vi "NI 5772 (AC) - TIS Mode Enabled (FPGA)Original.vi"() -> ()   [LabVIEW 2020]
doc: "Example Description:\nThis example demonstrates how to enable Time Interleaved Sampling with the NI 5772 adapter module to achieve a sampling rate of 1.6GS/s. This example continuously acquires records of analog input data from the NI 5772 adapter module. It allows you to select an AI channel, trigger type, and record size. This VI must be compiled before it is run. \n\nRunning the VI:\nThis VI must be run from the NI 5772 - Getting Started (Host).vi. Refer to the host VI documentation for steps regarding running and configuring the FPGA VI. \n\nExecution Steps:\nRefer to the Block Diagram of this VI for execution comments."
uses:
  D:/Program_Files/Labview2018/LabVIEW 2020/examples/FlexRIO/IO Modules/NI 5772/NI 5772 (AC) - TIS Mode Enabled/Controls/AI Trigger Type.ctl
  D:/Program_Files/Labview2018/LabVIEW 2020/examples/FlexRIO/IO Modules/NI 5772/NI 5772 (AC) - TIS Mode Enabled/Controls/Aquire State.ctl
  <vilib>/Platform/TimedLoop/XDataNode/timing_clust.ctl
  <vilib>/Platform/TimedLoop/XDataNode/nitl_modes.ctl
  <vilib>/Platform/TimedLoop/XDataNode/wakeup.ctl
  <vilib>/rvi/Emulation/niFpgaGetClockAttributes.vi
  <vilib>/rvi/Emulation/niFpgaSctlEmulationGetInTimedLoop.vi
  <vilib>/rvi/Emulation/niFpgaEmulationReportErrorSimple.vi
  <vilib>/rvi/eio/common/nirviEmuTemplateMethod_errors.vi
  <vilib>/rvi/Emulation/niFpgaCriticalErrorInLSC.vi
  <vilib>/rvi/Emulation/niFpgaEmulationIsFPGAContextNoSignature.vi
  <vilib>/rvi/errors/niFpgaSetErrorForExecOnDevCompSimple.vi
  <vilib>/rvi/eio/common/nirviEmuReportErrorAndStop.vi
  <vilib>/rvi/DataTransferAndStorage/Container/Common/niFpgaContainerGetUniqueNameForEmu.vi
  <vilib>/rvi/FIFO/Fifo_Resource/nirvififoEmulationSetSize.vi
  <vilib>/rvi/FIFO/Fifo_Resource/nirviFifoEmulationQueueMgr.vi
  <instcachedir>/0/nirviFifoEmulationQueueMgr_E5CAEC123FF24DC58D834DCA3CDAA9B5.lvgen/nirviFifoEmulationQueueMgr_E5CAEC123FF24DC58D834DCA3CDAA9B5_000.vi
  <vilib>/Utility/error.llb/Clear Errors.vi
  <vilib>/rvi/FIFO/Fifo_Resource/nirvififoEmulationCreateLock.vi
  <vilib>/rvi/Emulation/niFpgaProcessEmulError.vi
  <vilib>/rvi/FIFO/Fifo_Resource/nirvififoEmulationObtainLock.vi
  <vilib>/rvi/FIFO/Fifo_Resource/nirvififoEmulationReleaseLock.vi
  <vilib>/rvi/occurrence/nirviWaitOnOccurrenceBase.vi
  <vilib>/rvi/errors/nirviReportUnexpectedCaseInternalError.vi
  <vilib>/rvi/errors/nirviReportUnexpectedCaseInternalError (U32).vi
  <vilib>/rvi/interface/RandomDataEmulation/niFpgaRandomDataHandleErrors.vi
  <vilib>/rvi/FIFO/Fifo_Resource/nirvififoEmulationDetermineInputValidOut.vi
  <vilib>/eio/EIONode/EIONode.xnode
  <vilib>/Platform/TimedLoop/XDataNode/XDataNode.xnode
  <vilib>/rvi/DataTransferAndStorage/Container/XNode/niFpgaContainer.xnode
  <vilib>/rvi/FIFO/Fifo_Resource/nirvififoEmulationRead.vi
  <vilib>/rvi/interface/RandomDataEmulation/nirviRandomDataFpgaReadWriteTemplate.vi
  <vilib>/rvi/FIFO/Fifo_Resource/nirvififoEmulationWrite.vi
  <vilib>/Platform/TimedLoop/XDataNode/XDNodeRunTimeDep.lvlib
panel:
  out "TS FIFO In Overflow?":bool caption="FIFO Overflow?"
  in  "Samples Per Trigger":u16=512 min=1 step=1
  in  "Arm Trigger":bool
  in  "User Command Commit":bool
  in  "User Command":u8
  out "User Command Idle":bool
  out "User Command Status":u8
  in  "User Data 0":u16
  in  "User Data 1":u8
  out "PLL Locked":bool
  out "User Error":bool
  out "Configured?":bool
  out "DMA FIFO Overflow?":bool caption="FIFO Overflow?"
  in  "Trigger Level":i16
  in  "Trigger Type":T1
  # "Resource Configuration"
  # "Refer to the Block Diagram of this VI for execution comments."
  # "For other instructions, select Help>>Show Context Help and move the cursor over the VI icon to display help for this VI."
  # "Analog Input"
  # "Clock Configuration"
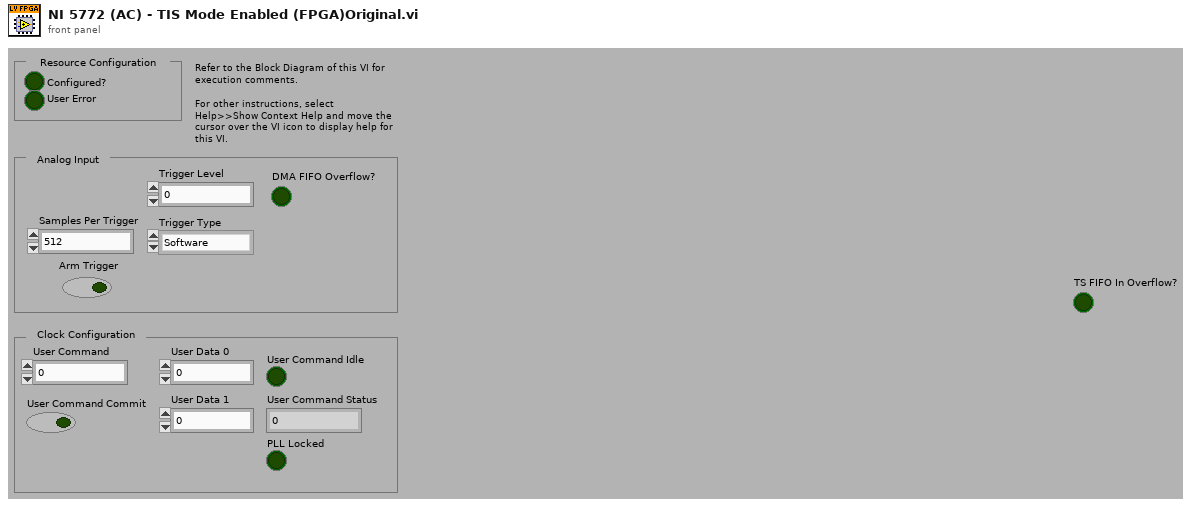
[diagram p1: front panel]
types:
  T1 = typedef "AI Trigger Type.ctl" = enum8{"Software", "Data Edge"}
  T2 = typedef "Aquire State.ctl" = enum8{"Idle", "Wait for Trigger", "Acquire"}
  T3 = typedef "XDNodeRunTimeDep.lvlib/timing_clust.ctl" = cluster{"Expected End [f-1]":u64, "Actual End [f-1]":u64, "Finished Late? [f-1]":bool, "Expected End [i-1]":u64, "Actual End [i-1]":u64, "Finished Late? [i-1]":bool, "Expected Start [i]":u64, "Actual Start [i]":u64, "Expected Start [f]":u64, "Actual Start [f]":u64, "Source Name":string, "Structure Name":string, "Period":i64, "Deadline":i64, "Offset":i64, "Start":i64, "Priority":i32, "Timeout":i32, "Mode":T4, "Wakeup Reason":T5, "Error":errorcluster, "Source Type":string, "Secondary Source Type":string, "Global End Time":u64, "Global Start Time":u64, "Frame Duration":u64, "Iteration Duration":u64, "Assigned CPU":i32, "I/O Scan Engine Mode":u32}
  T4 = typedef "XDNodeRunTimeDep.lvlib/nitl_modes.ctl" = enum32{"No Change", "Process missed periods, maintain original phase", "Discard missed periods, maintain original phase", "Process missed periods, ignore original phase", "Discard missed periods, ignore original phase"}
  T5 = typedef "XDNodeRunTimeDep.lvlib/wakeup.ctl" = enum32{"Normal", "Aborted", "Asynchronous wakeup", "Timing source error", "Timed loop error", "Timeout"}
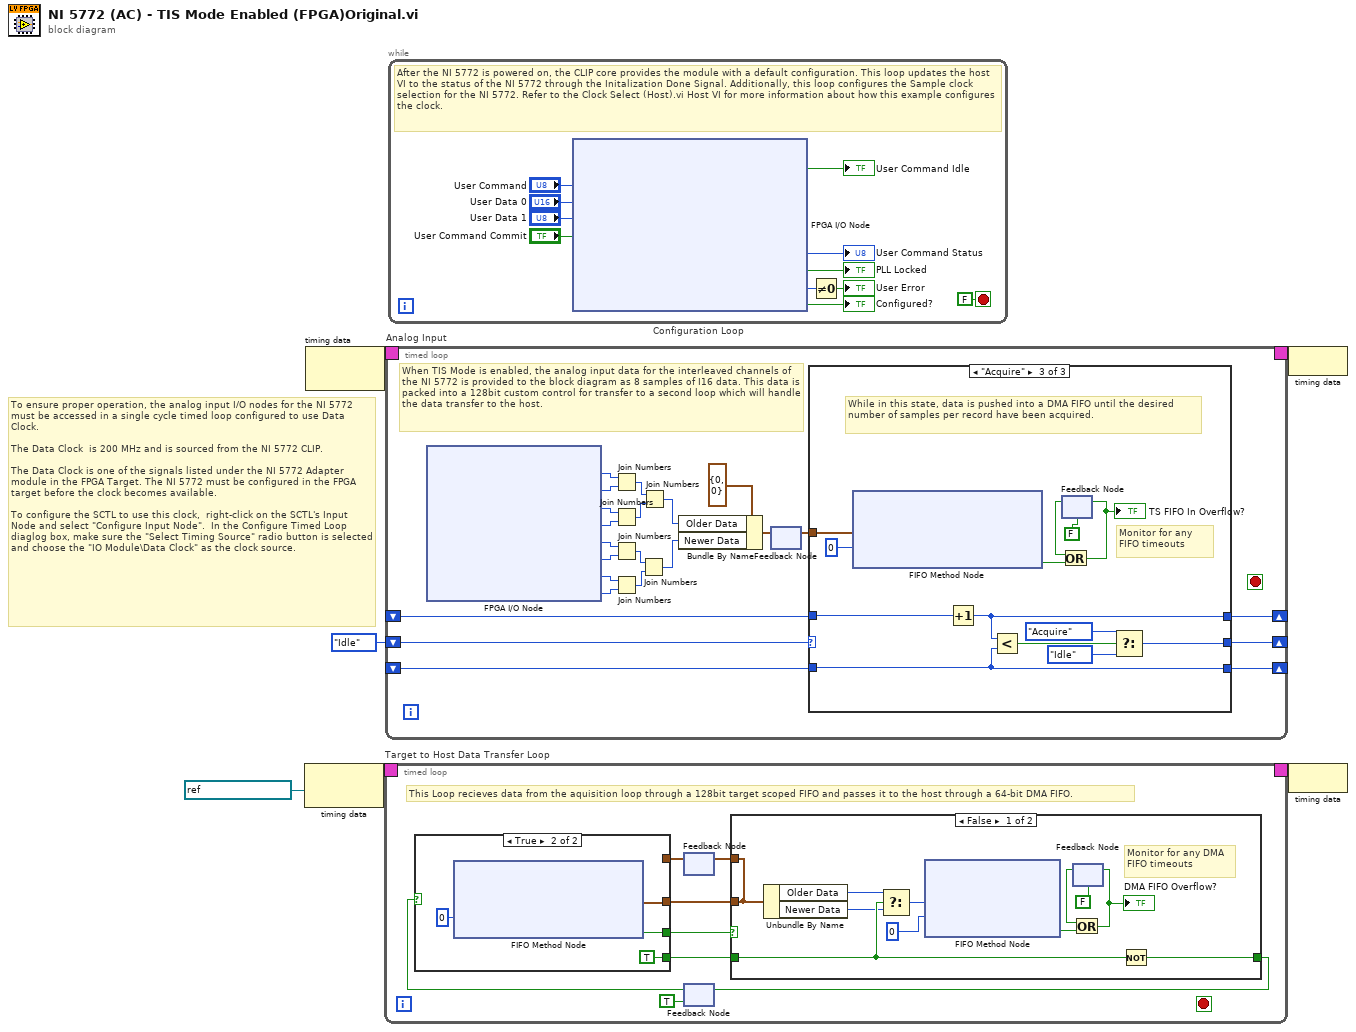
[diagram p0: block diagram]
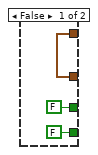
[diagram p2: hidden frame]
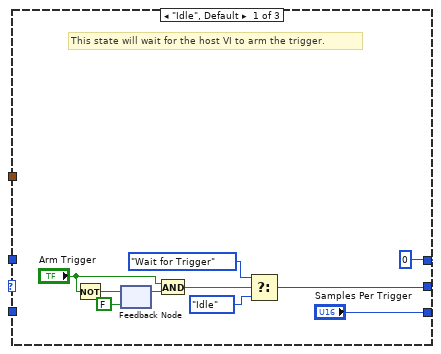
[diagram p4: hidden frame]
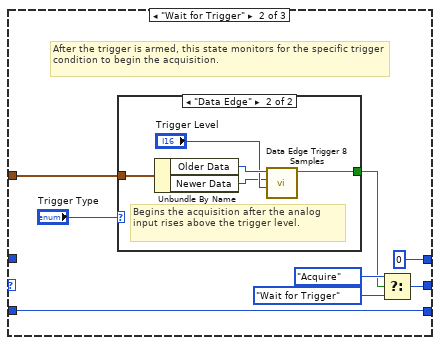
[diagram p5: hidden frame]
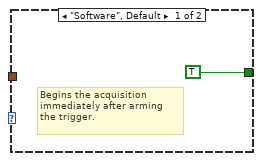
[diagram p6: hidden frame]
diagram:
  # "To ensure proper operation, the analog input I/O nodes for the NI 5772 must be accessed in a single cycle timed loop configured to use Data Clock. \n\nThe Data Clock  is 200 MHz and is sourced from the NI 5772 CLIP.\n\nThe Data Clock is one of the signals listed under the NI 5772 Adapter module in the FPGA Target. The NI 5772 must be configured in the FPGA target before the clock becomes available. \n\nTo configure the SCTL to use this clock,  right-click on the SCTL's Input Node and select \"Configure Input Node\".  In the Configure Timed Loop diaglog box, make sure the \"Select Timing Source\" radio button is selected and choose the \"IO Module\\Data Clock\" as the clock source."
  n1 = node-c288(refnum<k21> "100 MHz Clock" ("Source Name")) -> (w4:T3)
  n2 = node-c288() -> (w6:T3)  [unwired: 1 in]
  n3 = timed-loop "Target to Host Data Transfer Loop" {
    timing: w4 -> [_]
    timing-out: [_] -> w3
    stop <- _ stop-if-true
    # "This Loop recieves data from the aquisition loop through a 128bit target scoped FIFO and passes it to the host through a 64-bit DMA FIFO."
    n4 = feedback #1() -> (w11:cluster{"Older Data":u64, "Newer Data":u64})  [unwired: 1 in]
    n5 = feedback #2(TRUE ("Timed Out?")) -> (w12:bool)
    n6 = case shown="True" w12 {
      tunnel: [w15 w18] -> w9
      tunnel: [FALSE ("Timed Out?") w19] -> w8
      tunnel: [FALSE ("Timed Out?") TRUE ("Timed Out?")] -> w7
      tunnel: w11 -> [w15 _]
      frame False {
      }
      frame True {
        n7 = xnode ("FIFO Method Node")("Timeout"=0) -> ("Element"=w18:cluster{"Older Data":u64, "Newer Data":u64}, "Timed Out?"=w19:bool)  [unwired: 1 in, 1 out]
      }
    }
    n8 = case shown="False" w8 {
      tunnel: [w27 w34] -> w13
      tunnel: w7 -> [w28 w34]
      tunnel: w9 -> [w26 w33]
      tunnel: [w26 w33] -> w10
      frame False {
        # "Monitor for any DMA FIFO timeouts"
        n9 = Unbundle By Name(w26) -> ("Older Data"=w29:u64, "Newer Data"=w22:u64)
        n10 = Select(t=w29, s=w28, f=w22) -> (s? t:f=w24:u64)
        n11 = xnode ("FIFO Method Node")("Element"=w24, "Timeout"=0) -> ("Timed Out?"=w25:bool)  [unwired: 1 in, 1 out]
        n12 = feedback #3(FALSE) -> (w32:bool)
        n13 = Or(x=w32, y=w25) -> (x .or. y?=w30:bool)
        "DMA FIFO Overflow?" <- w30
        n14 = feedback-in #3(w30) -> ()
        n15 = Not(x=w28) -> (.not. x?=w27:bool)
      }
      frame True {
      }
    }
    n16 = feedback-in #1(w10) -> ()
    n17 = feedback-in #2(w13) -> ()
  }
  n18 = timed-loop "Analog Input" {
    timing: w6 -> [_]
    timing-out: [_] -> w5
    shift-right: [w58] -> _
    shift-left: Aquire_State."Idle" ("Acquire State") -> [w48]
    shift-right: [w59] -> _
    shift-left: _ -> [w49]
    shift-right: [w57] -> _
    shift-left: _ -> [w47]
    stop <- _ stop-if-true
    # "When TIS Mode is enabled, the analog input data for the interleaved channels of the NI 5772 is provided to the block diagram as 8 samples of I16 data. This data is packed into a 128bit custom control for transfer to a second loop which will handle the data transfer to the host."
    n19 = xnode "FPGA I/O Node"() -> ("IO Module\\AI 1 Data N-3"=w40:i16, "IO Module\\AI 0 Data N-3"=w39:i16, "IO Module\\AI 1 Data N-2"=w38:i16, "IO Module\\AI 0 Data N-2"=w37:i16, "IO Module\\AI 1 Data N-1"=w41:i16, "IO Module\\AI 0 Data N-1"=w42:i16, "IO Module\\AI 1 Data N"=w43:i16, "IO Module\\AI 0 Data N"=w44:i16)  [unwired: 8 in, 8 out]
    n20 = Join Numbers(hi=w40, lo=w39) -> ((hi.lo)=w52:u32)
    n21 = Join Numbers(hi=w38, lo=w37) -> ((hi.lo)=w54:u32)
    n22 = Join Numbers(hi=w41, lo=w42) -> ((hi.lo)=w53:u32)
    n23 = Join Numbers(hi=w43, lo=w44) -> ((hi.lo)=w55:u32)
    n24 = Join Numbers(hi=w53, lo=w55) -> ((hi.lo)=w45:u64)
    n25 = Join Numbers(hi=w52, lo=w54) -> ((hi.lo)=w46:u64)
    n26 = Bundle By Name(cluster=cluster{"Older Data":u64, "Newer Data":u64} {"Older Data"=0, "Newer Data"=0} ("Element"), "Older Data"=w46, "Newer Data"=w45) -> (w50:cluster{"Older Data":u64, "Newer Data":u64})
    n27 = feedback #4() -> (w56:cluster{"Older Data":u64, "Newer Data":u64})  [unwired: 1 in]
    n28 = feedback-in #4(w50) -> ()
    n29 = case shown="\"Acquire\"" w48 {
      tunnel: [u16 0 u16 0 w96] -> w59
      tunnel: w49 -> [_ _ w95]
      tunnel: [w62 w72 w93] -> w58
      tunnel: ["Samples Per Trigger" w76 w90] -> w57
      tunnel: w47 -> [_ w76 w90]
      tunnel: w56 -> [_ w75 w89]
      frame "Idle", Default {
        # "This state will wait for the host VI to arm the trigger."
        n30 = Not(x="Arm Trigger") -> (.not. x?=w69:bool)
        n31 = feedback #5(FALSE) -> (w68:bool)
        n32 = feedback-in #5(w69) -> ()
        n33 = And(x="Arm Trigger", y=w68) -> (x .and. y?=w64:bool)
        n34 = Select(t=Aquire_State."Wait for Trigger" ("Acquire State"), s=w64, f=Aquire_State."Idle" ("Acquire State")) -> (s? t:f=w62:T2)
      }
      frame "Wait for Trigger" {
        # "After the trigger is armed, this state monitors for the specific trigger condition to begin the acquisition."
        n35 = case shown="\"Data Edge\"" "Trigger Type" {
          tunnel: w75 -> [_ w83]
          tunnel: [TRUE ("Trigger") w82] -> w70
          frame "Software", Default {
            # "Begins the acquisition immediately after arming the trigger."
          }
          frame "Data Edge" {
            # "Begins the acquisition after the analog input rises above the trigger level."
            n36 = Unbundle By Name(w83) -> ("Older Data"=w81:u64, "Newer Data"=w79:u64)
            n37 = call "Data Edge Trigger 8 Samples.vi"("Trigger Level"="Trigger Level", "Newer Data In"=w79, "Older Data In"=w81) -> ("Trigger"=w82:bool)  [unwired: 8 in]
          }
        }
        n38 = Select(t=Aquire_State."Acquire" ("Acquire State"), s=w70, f=Aquire_State."Wait for Trigger") -> (s? t:f=w72:T2)
      }
      frame "Acquire" {
        # "Monitor for any  FIFO timeouts"
        # "While in this state, data is pushed into a DMA FIFO until the desired number of samples per record have been acquired."
        n39 = xnode ("FIFO Method Node")("Element"=w89, "Timeout"=0) -> ("Timed Out?"=w84:bool)  [unwired: 1 in, 1 out]
        n40 = Increment(x=w95) -> (x+1=w96:u16)
        n41 = Less?(x=w96, y=w90) -> (x < y?=w94:bool)
        n42 = feedback #6(FALSE) -> (w85:bool)
        n43 = Or(x=w85, y=w84) -> (x .or. y?=w86:bool)
        "TS FIFO In Overflow?" <- w86
        n44 = feedback-in #6(w86) -> ()
        n45 = Select(t=Aquire_State."Acquire" ("Acquire State"), s=w94, f=Aquire_State."Idle" ("Acquire State")) -> (s? t:f=w93:T2)
      }
    }
  }
  n46 = while "Configuration Loop" {
    stop <- FALSE stop-if-true
    # "After the NI 5772 is powered on, the CLIP core provides the module with a default configuration. This loop updates the host VI to the status of the NI 5772 through the Initalization Done Signal. Additionally, this loop configures the Sample clock selection for the NI 5772. Refer to the Clock Select (Host).vi Host VI for more information about how this example configures the clock."
    n47 = xnode "FPGA I/O Node"("IO Module\\User Command"="User Command", "IO Module\\User Data 0"="User Data 0", "IO Module\\User Data 1"="User Data 1", "IO Module\\User Command Commit"="User Command Commit") -> ("IO Module\\User Command Idle"=→"User Command Idle":bool, "IO Module\\User Command Status"=→"User Command Status":u8, "IO Module\\PLL Locked"=→"PLL Locked":bool, "IO Module\\User Error"=w104:u8, "IO Module\\Initialization Done"=→"Configured?":bool)  [unwired: 9 in, 9 out]
    n48 = Not Equal To 0?(x=w104) -> (x != 0?=→"User Error":bool)
  }
  n49 = node-c288(w5) -> ()
  n50 = node-c288(w3) -> ()
